vi "AWG Calculate Gain Offset from VHi Vlo.vi"(8 "AmpGain":dbl=15.0 format="%#_13g", 10 "Vlo":dbl=-1.0, 11 "VHi":dbl=1.0) -> (1 "Vrng":dbl, 2 "Offset":dbl, 3 "Gain":dbl)   [LabVIEW 2013]
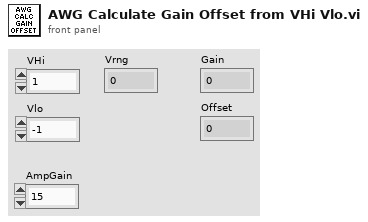
[diagram p1: front panel]
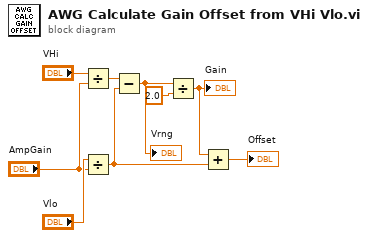
[diagram p0: block diagram]
diagram:
  n1 = Divide(x="VHi", y="AmpGain") -> (x/y=w4:dbl)
  n2 = Divide(x="Vlo", y="AmpGain") -> (x/y=w1:dbl)
  n3 = Subtract(x=w4, y=w1) -> (x-y=w9:dbl)
  "Vrng" <- w9
  n4 = Divide(x=w9, y=2.0) -> (x/y=w7:dbl)
  "Gain" <- w7
  n5 = Add(x=w7, y=w1) -> (x+y=→"Offset":dbl)
